vi "MD5Checksum_format_output.vi"(8 "s4":u32 format="%.0x", 9 "s3":u32 format="%.0x", 10 "s2":u32 format="%.0x", 11 "s1":u32 format="%.0x") -> (2 "MD5 message-digest (ASCII)":string, 3 "MD5 message-digest (HEX)":string)   [LabVIEW 2021, in "vi_lib.lvlib"]
doc: "This VI performs certain bitwise operations on the state variables and converts them to hex strings such that they can be concatenated and displayed as the MD5 message-digest."
uses:
  vi_lib.lvlib
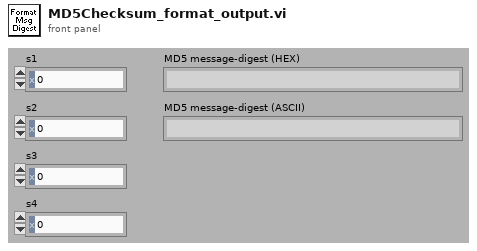
[diagram p1: front panel]
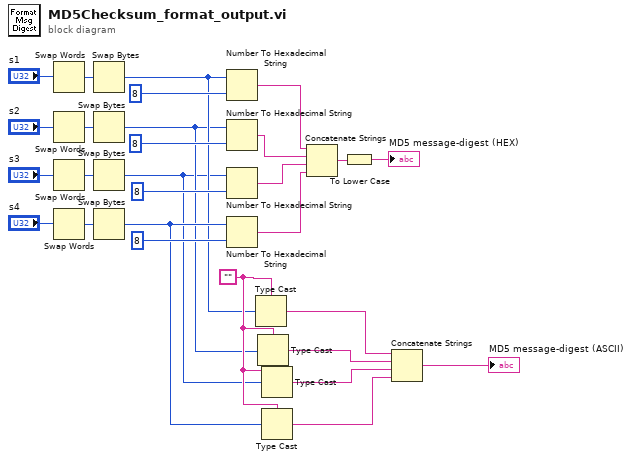
[diagram p0: block diagram]
diagram:
  w9 = "" ("MD5 message-digest 2")
  n1 = Swap Words(1:"s1") -> (0:w26:u32)
  n2 = Swap Words(1:"s2") -> (0:w25:u32)
  n3 = Swap Words(1:"s3") -> (0:w21:u32)
  n4 = Swap Words(1:"s4") -> (0:w19:u32)
  n5 = Swap Bytes(anything=w26) -> (byte swapped=w8:u32)
  n6 = Swap Bytes(anything=w25) -> (byte swapped=w7:u32)
  n7 = Swap Bytes(anything=w21) -> (byte swapped=w6:u32)
  n8 = Swap Bytes(anything=w19) -> (byte swapped=w10:u32)
  n9 = Number To Hexadecimal String(1:i16 8 ("width (-)"), 2:w8) -> (0:w16:string)
  n10 = Number To Hexadecimal String(1:i16 8 ("width (-)"), 2:w7) -> (0:w15:string)
  n11 = Number To Hexadecimal String(1:i16 8 ("width (-)"), 2:w6) -> (0:w14:string)
  n12 = Number To Hexadecimal String(1:i16 8 ("width (-)"), 2:w10) -> (0:w13:string)
  n13 = Type Cast(type=w9, x=w8) -> (*(type *) &x=w5:string)
  n14 = Type Cast(type=w9, x=w7) -> (*(type *) &x=w4:string)
  n15 = Type Cast(type=w9, x=w6) -> (*(type *) &x=w3:string)
  n16 = Type Cast(type=w9, x=w10) -> (*(type *) &x=w2:string)
  n17 = Concatenate Strings(w16, w15, w14, w13) -> (w12:string)
  n18 = To Lower Case(string=w12) -> (all lower case string=→"MD5 message-digest (HEX)":string)
  n19 = Concatenate Strings(w5, w4, w3, w2) -> (→"MD5 message-digest (ASCII)":string)
